vi "NewDataAdded Event Callback.vi"(4 "New Curve Values":T1, 5 "Event Data":cluster{"sender":refnum<k24>, "e":refnum<k24>}, 6 "Control Ref":refnum<k24>, 7 "Event Common Data":T2) -> ()   [LabVIEW 2025]
uses:
  E:/PSCode/PalmSens_SDK/labview/PalmSens/Libraries/PalmSens.Core.Simplified.LabVIEW.dll
  Libraries/PalmSens.Core.Simplified.LabVIEW.dll
  NewCurveDataEventArgs.ctl
  LiveCurveResult.ctl
  MeasurementsResult.ctl
  MeasurementResults.ctl
  CurvesByMeasurement.ctl
  MeasurementInfo.ctl
  CurveInfo.ctl
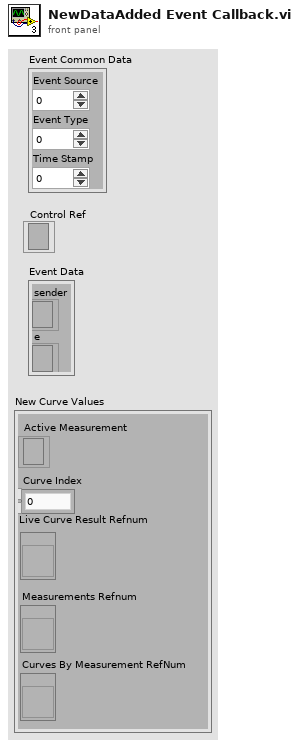
[diagram p1: front panel]
types:
  T1 = typedef "NewCurveDataEventArgs.ctl" = cluster{"Active Measurement":refnum<k24>, "Live Curve Result Refnum":refnum<vi>, "Measurements Refnum":refnum<vi>, "Curves By Measurement RefNum":refnum<vi>, "Curve Index":i32}
  T2 = cluster{"Event Source":i32, "Event Type":u32, "Time Stamp":u32}
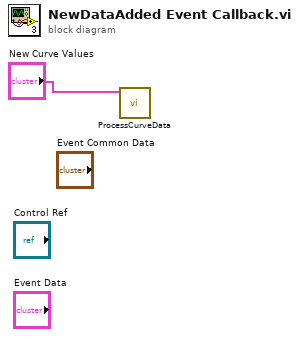
[diagram p0: block diagram]
diagram:
  n1 = call "ProcessCurveData.vi"("New Curve Values"="New Curve Values") -> ()  [unwired: 11 in]
